vi "CVT.vi"(7 "Action":T1, 8 "error in (no error)":errorcluster, 10 "Value in":variant, 11 "Key":string) -> (0 "error out":errorcluster, 2 "Replaced?/Found?":bool, 3 "Value out":variant)   [LabVIEW 2017, in "Toolbox.lvlib"]
uses:
  Toolbox.lvlib
  Control/CVT Action.ctl
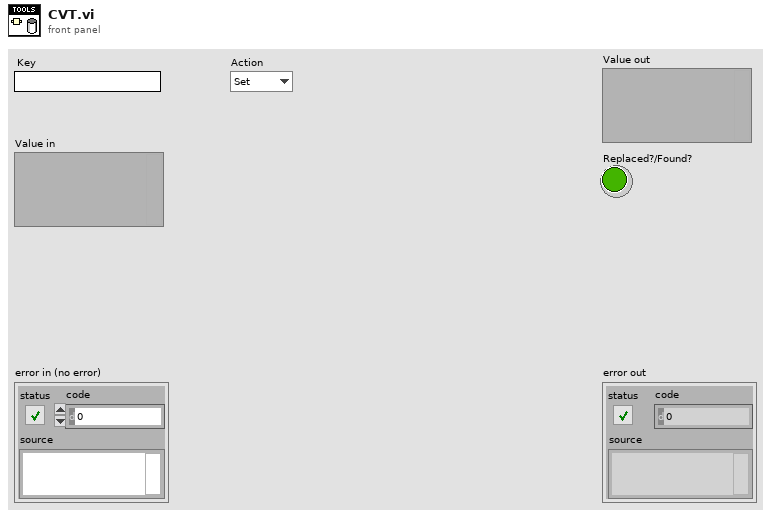
[diagram p1: front panel]
types:
  T1 = typedef "Toolbox.lvlib/CVT Action.ctl" = enum16{"Set", "Replace", "Get", "Check", "Delete", "Delete All"}
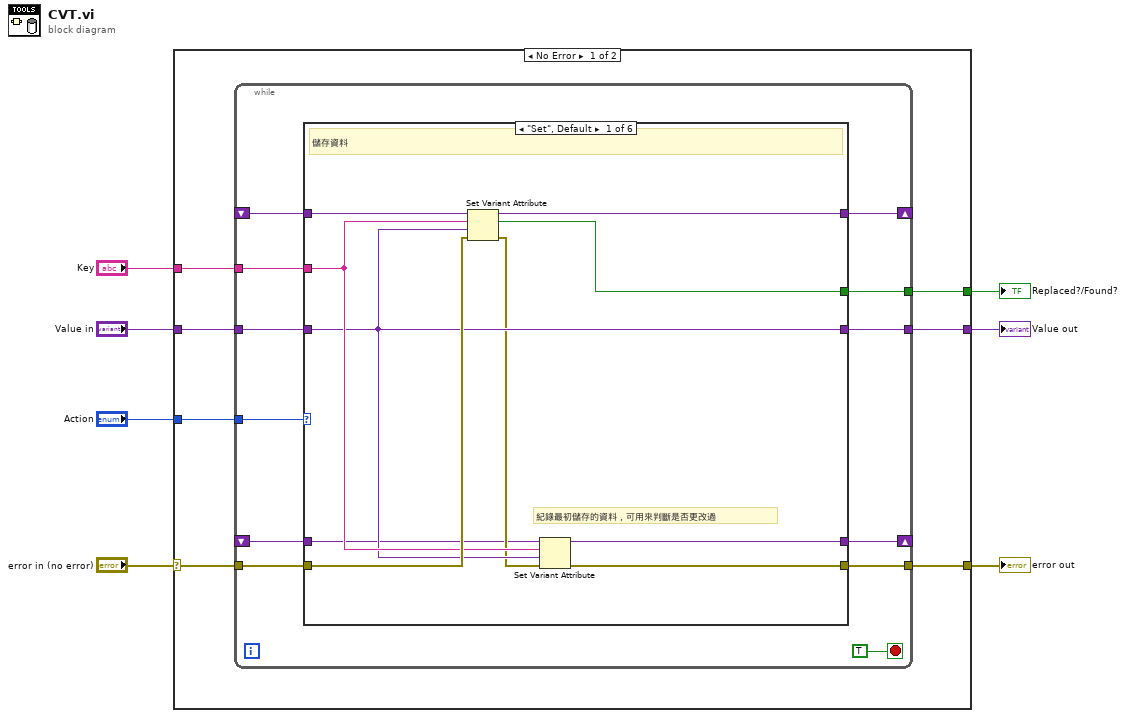
[diagram p0: block diagram]
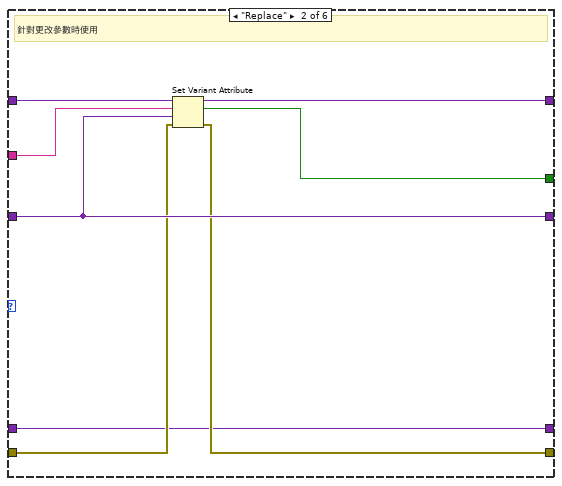
[diagram p2: hidden frame]
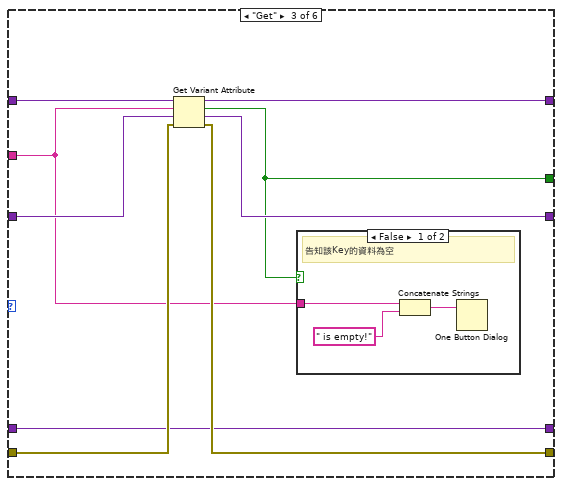
[diagram p3: hidden frame]
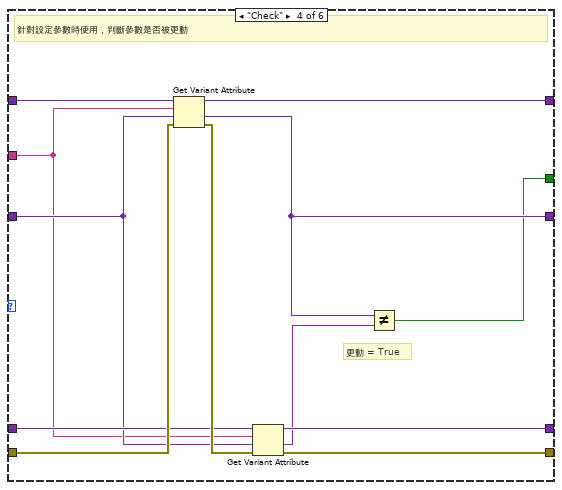
[diagram p5: hidden frame]
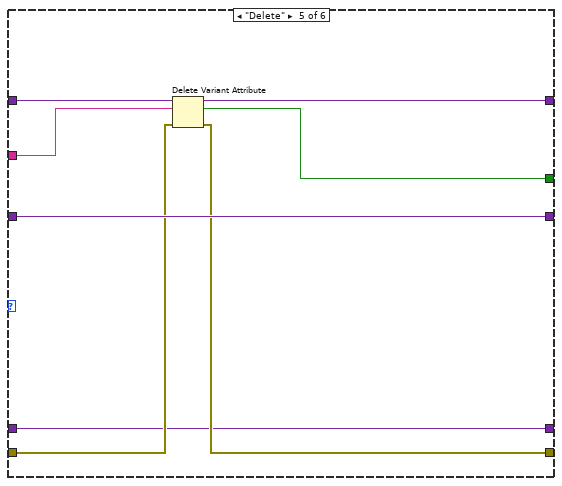
[diagram p6: hidden frame]
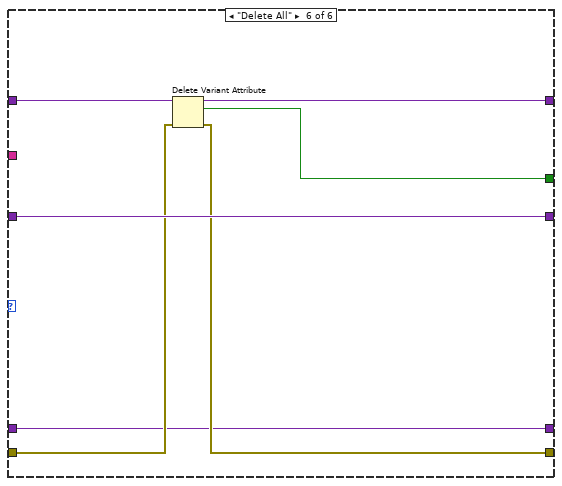
[diagram p7: hidden frame]
diagram:
  n1 = case shown="No Error" "error in (no error)" {
    selector: "error in (no error)" -> [w10 w84]
    tunnel: "Value in" -> [w14 w85]
    tunnel: "Action" -> [w13 _]
    tunnel: "Key" -> [w12 _]
    tunnel: [w9 w84] -> w2
    tunnel: [w11 w85] -> w3
    tunnel: [w8 _] -> w1
    frame No Error {
      n2 = while {
        tunnel: w13 -> [w25]
        tunnel: w12 -> [w24]
        shift-right: [w23] -> _
        shift-left: _ -> [w22]
        tunnel: w14 -> [w26]
        tunnel: [w21] -> w11
        tunnel: w10 -> [w19]
        tunnel: [w18] -> w9
        tunnel: [w17] -> w8
        shift-right: [w16] -> _
        shift-left: _ -> [w15]
        stop <- TRUE stop-if-true
        n3 = case shown="\"Set\", Default" w25 {
          tunnel: w26 -> [w31 w41 w53 w61 w73 w81]
          tunnel: w24 -> [w32 w42 w46 w60 w74 _]
          tunnel: [w36 w44 w52 w68 w76 w83] -> w23
          tunnel: w22 -> [w35 w43 w51 w67 w75 w82]
          tunnel: [w31 w41 w50 w58 w73 w81] -> w21
          tunnel: w19 -> [w34 w40 w49 w66 w72 w80]
          tunnel: [w30 w39 w48 w64 w71 w79] -> w18
          tunnel: [w33 w38 w47 w57 w70 w78] -> w17
          tunnel: [w28 w37 w45 w62 w69 w77] -> w16
          tunnel: w15 -> [w27 w37 w45 w63 w69 w77]
          frame "Set", Default {
            # "紀錄最初儲存的資料，可用來判斷是否更改過"
            # "儲存資料"
            n4 = Set Variant Attribute(Variant=w35, name=w32, value=w31, error in=w34) -> (Variant out=w36:variant, replaced=w33:bool, error out=w29:errorcluster)
            n5 = Set Variant Attribute(Variant=w27, name=w32, value=w31, error in=w29) -> (Variant out=w28:variant, error out=w30:errorcluster)  [unwired: 1 out]
          }
          frame "Replace" {
            # "針對更改參數時使用"
            n6 = Set Variant Attribute(Variant=w43, name=w42, value=w41, error in=w40) -> (Variant out=w44:variant, replaced=w38:bool, error out=w39:errorcluster)
          }
          frame "Get" {
            n7 = Get Variant Attribute(Variant=w51, name=w46, default value (empty Variant)=w53, error in=w49) -> (duplicate Variant=w52:variant, found=w47:bool, value=w50:variant, error out=w48:errorcluster)
            n8 = case shown="False" w47 {
              tunnel: w46 -> [w55 _]
              frame False {
                # "告知該Key的資料為空"
                n9 = Concatenate Strings(w55, " is empty!") -> (w56:string)
                n10 = One Button Dialog(message=w56) -> ()  [unwired: 1 in, 1 out]
              }
              frame True {
              }
            }
          }
          frame "Check" {
            # "更動 = True"
            # "針對設定參數時使用，判斷參數是否被更動"
            n11 = Get Variant Attribute(Variant=w67, name=w60, default value (empty Variant)=w61, error in=w66) -> (duplicate Variant=w68:variant, value=w58:variant, error out=w65:errorcluster)  [unwired: 1 out]
            n12 = Get Variant Attribute(Variant=w63, name=w60, default value (empty Variant)=w61, error in=w65) -> (duplicate Variant=w62:variant, value=w59:variant, error out=w64:errorcluster)  [unwired: 1 out]
            n13 = Not Equal?(x=w58, y=w59) -> (x != y?=w57:bool)
          }
          frame "Delete" {
            n14 = Delete Variant Attribute(4:w72, 6:w74, 7:w75) -> (0:w71:errorcluster, 2:w70:bool, 3:w76:variant)
          }
          frame "Delete All" {
            n15 = Delete Variant Attribute(4:w80, 7:w82) -> (0:w79:errorcluster, 2:w78:bool, 3:w83:variant)  [unwired: 1 in]
          }
        }
      }
    }
    frame Error {
    }
  }
  "Value out" <- w3
  "error out" <- w2
  "Replaced?/Found?" <- w1
